vi "Stop Core.vi"(10 "final error code":i32, 11 "LHW-TDMS-Storage-Actor in":refnum<class "LHW-TDMS-Storage-Actor.lvclass">) -> (3 "LHW-TDMS-Storage-Actor out":refnum<class "LHW-TDMS-Storage-Actor.lvclass">)   [LabVIEW 2016, in "LHW-TDMS-Storage.lvlib" / "LHW-TDMS-Storage-Actor.lvclass"]
doc: "(<B>Filename</B>: Actor Framework.lvlib:Actor.lvclass:Stop Core.vi)\n\nDefines what the actor does before it stops. Use the <B>final error code</B> input to determine whether the actor shut down in response to an error.\n\nBy default, this method does nothing. A descendant class may override it to define behavior, such as shutting down any processes the actor initiated in its override of the Actor Core method."
uses:
  LHW-TDMS-Storage-Actor.lvclass
  LHW-TDMS-Storage-Actor.lvclass/LHW-TDMS-Storage-Actor.ctl
  LHW-Storage/LHW-Storage-Actor.lvclass
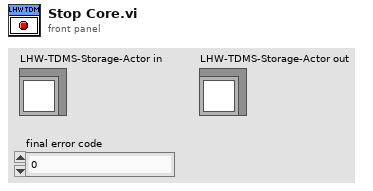
[diagram p1: front panel]
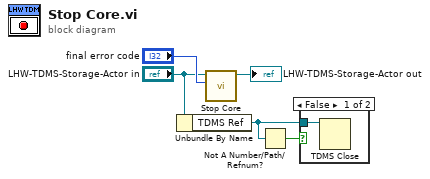
[diagram p0: block diagram]
diagram:
  n1 = Unbundle By Name("LHW-TDMS-Storage-Actor in") -> ("TDMS Ref"=w2:refnum<k34>)
  n2 = call-parent "Stop Core.vi"("final error code"="final error code", "Actor in"="LHW-TDMS-Storage-Actor in") -> ("Actor out"=→"LHW-TDMS-Storage-Actor out":refnum<class "LHW-TDMS-Storage-Actor.lvclass">)  [unwired: 9 in]
  n3 = Not A Number/Path/Refnum?(number/path/refnum=w2) -> (NaN/Path/Refnum?=w1:bool)
  n4 = case shown="False" w1 {
    tunnel: w2 -> [w6 _]
    frame False {
      n5 = TDMS Close(11:w6) -> ()  [unwired: 1 in, 2 out]
    }
    frame True {
    }
  }
